vi "XML Script - Wires.vi"(3 "destinations":string[](array[string]), 4 "source":string) -> (1 "source (dup)":string, 2 "XML":string)   [LabVIEW 2020]
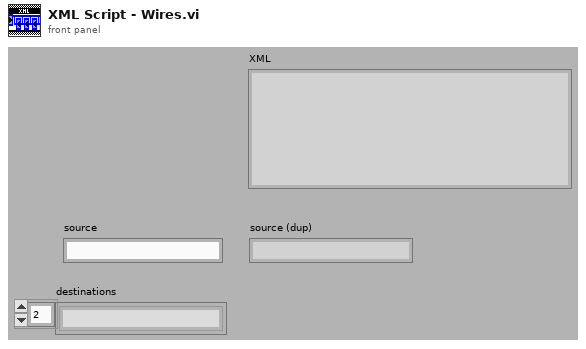
[diagram p1: front panel]
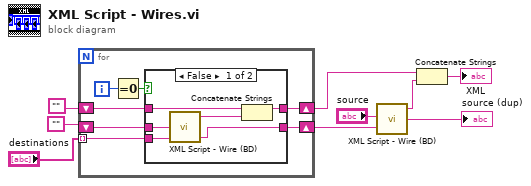
[diagram p0: block diagram]
diagram:
  n1 = for {
    shift-right: [w11] -> w6
    shift-left: "" -> [w10]
    tunnel: "destinations" -> [w14] mode=indexing
    shift-right: [w13] -> w4
    shift-left: "" -> [w12]
    i -> [w15]
    n2 = Equal To 0?(x=w15) -> (x = 0?=w16:bool)
    n3 = case shown="False" w16 {
      tunnel: w14 -> [w22 w24]
      tunnel: [w17 w24] -> w13
      tunnel: w12 -> [w21 _]
      tunnel: [w19 w23] -> w11
      tunnel: w10 -> [w18 w23]
      frame False {
        n4 = call <vilib>:"XML Script - Wire (BD).vi"("destination"=w22, "source"=w21) -> ("destination (dup)"=w17:string, "XML Script Command - Wire"=w20:string)  [unwired: 1 in, 1 out]
        n5 = Concatenate Strings(w18, w20) -> (w19:string)
      }
      frame True {
      }
    }
  }
  n6 = call <vilib>:"XML Script - Wire (BD).vi"("destination"=w4, "source"="source") -> ("source (dup)"=→"source (dup)":string, "XML Script Command - Wire"=w3:string)  [unwired: 1 in, 1 out]
  n7 = Concatenate Strings(w6, w3) -> (→"XML":string)
